vi "VoltageInputSetVoltageRange.vi"(0 "error in (no error)":errorcluster, 2 "Voltage Range":u32(ring) items=["VOLTAGE_RANGE_10mV"=1, "VOLTAGE_RANGE_40mV"=2, "VOLTAGE_RANGE_200mV"=3, "VOLTAGE_RANGE_312_5mV"=4, "VOLTAGE_RANGE_400mV"=5, "VOLTAGE_RANGE_1000mV"=6, "VOLTAGE_RANGE_2V"=7, "VOLTAGE_RANGE_5V"=8, "VOLTAGE_RANGE_15V"=9, "VOLTAGE_RANGE_40V"=10, "VOLTAGE_RANGE_AUTO"=11], 3 "Device In":u64) -> (7 "error out":errorcluster, 10 "Device Out":u64)   [LabVIEW 2012, in "Phidget Voltage Input.lvlib"]
doc: "${VoltageRange:Header}"
uses:
  <instrlib>/Phidgets/Phidget Voltage Input/Phidget Voltage Input.lvlib
  <instrlib>/Phidgets/Phidget Common/Phidget Common.lvlib
  phidget22.dll
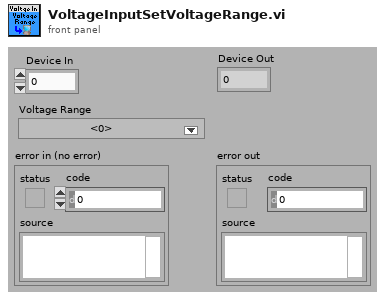
[diagram p1: front panel]
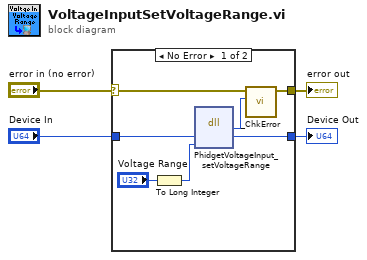
[diagram p0: block diagram]
diagram:
  n1 = case shown="No Error" "error in (no error)" {
    selector: "error in (no error)" -> [w9 w13]
    tunnel: [w8 w13] -> w3
    tunnel: "Device In" -> [w11 w12]
    tunnel: [w10 w12] -> w1
    frame No Error {
      n2 = To Long Integer(number="Voltage Range") -> (32bit integer=w5:i32)
      n3 = dll-call lib="phidget22.*" fn="PhidgetVoltageInput_setVoltageRange"("phid"=w11, "interval"=w5) -> ("return type"=w7:i32, "phid"=w10:u64)  [unwired: 4 in, 2 out]
      n4 = call <instrlib>:"_ChkError.vi"("Return Code"=w7, "error in (no error)"=w9) -> ("error out"=w8:errorcluster)  [unwired: 9 in]
    }
    frame Error {
    }
  }
  "error out" <- w3
  "Device Out" <- w1
